vi "Shooter_Test.vi"(1 "Joystick_IN":T1) -> ()   [LabVIEW 2020]
uses:
  Utility VIs/Joystick_Controls.ctl
  Systems/Shooter/Determiner/Shooter_Cluster.ctl
  Systems/Shooter/Determiner/Shooter_Control_States.ctl
  Systems/Shooter/Determiner/Shooter_Globals.vi
panel:
  in  "use this value":bool
  in  "power_flywheel":dbl
  in  "Power_Cowl":dbl=0.2 format="%#_13g"
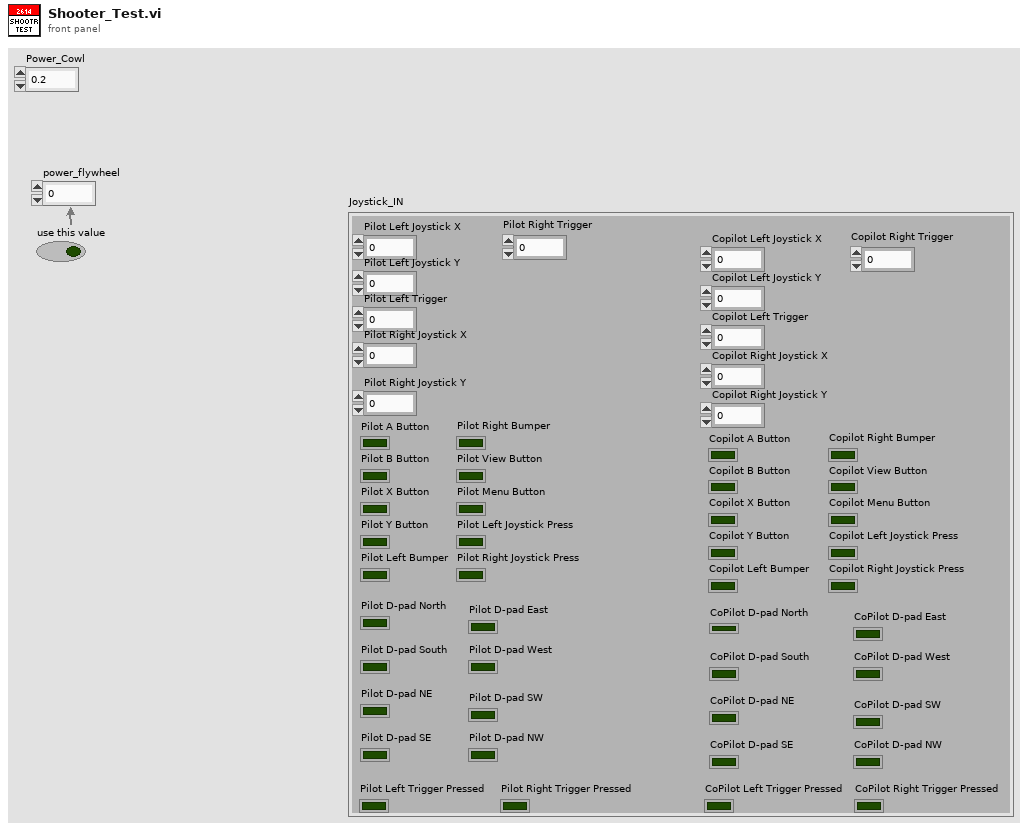
[diagram p1: front panel]
types:
  T1 = typedef "Joystick_Controls.ctl" = cluster{"Pilot Left Joystick X":dbl, "Pilot Left Joystick Y":dbl, "Pilot A Button":bool, "Pilot B Button":bool, "Pilot X Button":bool, "Pilot Y Button":bool, "Pilot Left Bumper":bool, "Pilot Right Bumper":bool, "Pilot View Button":bool, "Pilot Menu Button":bool, "Pilot Left Joystick Press":bool, "Pilot Right Joystick Press":bool, "Pilot Left Trigger":dbl, "Pilot Right Joystick X":dbl, "Pilot Right Joystick Y":dbl, "Pilot Right Trigger":dbl, "Copilot Left Joystick X":dbl, "Copilot Left Joystick Y":dbl, "Copilot A Button":bool, "Copilot B Button":bool, "Copilot X Button":bool, "Copilot Y Button":bool, "Copilot Left Bumper":bool, "Copilot Right Bumper":bool, "Copilot View Button":bool, "Copilot Menu Button":bool, "Copilot Left Joystick Press":bool, "Copilot Right Joystick Press":bool, "Copilot Left Trigger":dbl, "Copilot Right Joystick X":dbl, "Copilot Right Joystick Y":dbl, "Copilot Right Trigger":dbl, "Pilot D-pad North":bool, "Pilot D-pad South":bool, "Pilot D-pad East":bool, "Pilot D-pad West":bool, "Pilot D-pad NE ":bool, "Pilot D-pad SE":bool, "Pilot D-pad SW":bool, "Pilot D-pad NW":bool, "CoPilot D-pad North":bool, "CoPilot D-pad South":bool, "CoPilot D-pad East":bool, "CoPilot D-pad West":bool, "CoPilot D-pad NE":bool, "CoPilot D-pad SE":bool, "CoPilot D-pad SW":bool, "CoPilot D-pad NW":bool, "Pilot Left Trigger Pressed":bool, "Pilot Right Trigger Pressed":bool, "CoPilot Left Trigger Pressed":bool, "CoPilot Right Trigger Pressed":bool}
  T2 = typedef "Shooter_Cluster.ctl" = cluster{"Control_State":T3, "Shooting?":bool, "UpperGoal?":bool, "Limelight?":bool, "Flywheel_%Vbus":dbl, "Cowl_%Vbus":dbl, "Turret_%Vbus":dbl, "Parameters":dbl[], "Auto_Notifier":refnum<notifier>, "Step":i32, "Zero_Turret":bool, "Puke?":bool}
  T3 = typedef "Shooter_Control_States.ctl" = enum16{"No-Op", "Limelight_Shooting", "Shoot_From_Pose", "Test", "Command_Shoot", "Turret_Cowl_Zero", "Manual", "Puke-Op"}
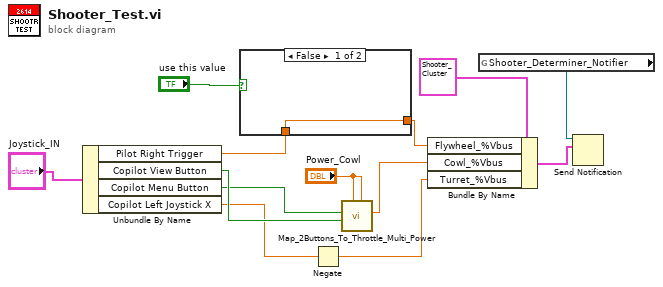
[diagram p0: block diagram]
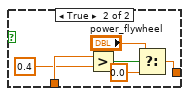
[diagram p2: hidden frame]
diagram:
  n1 = Unbundle By Name("Joystick_IN") -> ("Pilot Right Trigger"=w7:dbl, "Copilot View Button"=w6:bool, "Copilot Menu Button"=w5:bool, "Copilot Left Joystick X"=w2:dbl)
  n2 = case shown="False" "use this value" {
    tunnel: w7 -> [w14 w20]
    tunnel: [w14 w15] -> w9
    frame False {
    }
    frame True {
      n3 = Greater?(x=w20, y=0.4) -> (0:w18:bool)
      n4 = Select(t="power_flywheel", s=w18, f=0.0) -> (s? t:f=w15:dbl)
    }
  }
  n5 = Negate(x=w2) -> (-x=w1:dbl)
  n6 = call "Map_2Buttons_To_Throttle_Multi_Power.vi"("Power_Down"="Power_Cowl", "Power_Up"="Power_Cowl", "Down"=w6, "Up"=w5) -> ("Throttle"=w10:dbl)  [unwired: 7 in]
  n7 = Bundle By Name(cluster=T2 {"Control_State"=enum."No-Op", "Shooting?"=FALSE, "UpperGoal?"=FALSE, "Limelight?"=FALSE, "Flywheel_%Vbus"=0.0, "Cowl_%Vbus"=0.0, "Turret_%Vbus"=0.0, "Parameters"=[], "Auto_Notifier"=refnum, "Step"=0, "Zero_Turret"=FALSE, "Puke?"=FALSE} ("Shooter_Determiner"), "Flywheel_%Vbus"=w9, "Cowl_%Vbus"=w10, "Turret_%Vbus"=w1) -> (w12:T2)
  n8 = global read "Shooter_Globals.vi" "Shooter_Determiner_Notifier"() -> (w13:refnum<notifier>)
  n9 = Send Notification(notification=w12, notifier=w13) -> ()  [unwired: 1 in, 2 out]
